vi "Global_HW_Data Out.vi"() -> ()   [LabVIEW 2017, in "Gear.lvlib"]
uses:
  Gear.lvlib
panel:
  out "HW_Gear Present":bool
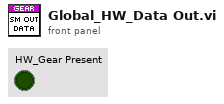
[diagram p1: front panel]
diagram:
